vi "etapa2.vi"() -> ()   [LabVIEW 2017]
uses:
  <vilib>/Analysis/baseanly.llb/Mean (DBL).vi
  <vilib>/MakerHub/LINX/Public/Utilities/Open Serial.vi
  <vilib>/measure/maspectr.llb/FFT Spectrum (Mag-Phase) for 1 Chan.vi
  <vilib>/MakerHub/LINX/LMH-LINX.lvlib
  <vilib>/Analysis/NI_AALBase.lvlib
  <vilib>/measure/NI_MAPro.lvlib
panel:
  out "Frequência predominante (Hz)":dbl
  in  "Loop":u8
  in  "Janela":u8
  out "Frequências":cluster{"f0":dbl, "df":dbl, "magnitude":dbl[]}(graph)
  out "Pontos adquiridos":waveform(dbl)(graph)
  out "Dup Command Number":u16
  out "Tempo entre medidas":u8[](array[numeric])
  out "Device Name":string
  in  "Serial Port":refnum<visa-resource-name>="N/A"
  in  "Baud Rate Override":u32
  # "Aquisição"
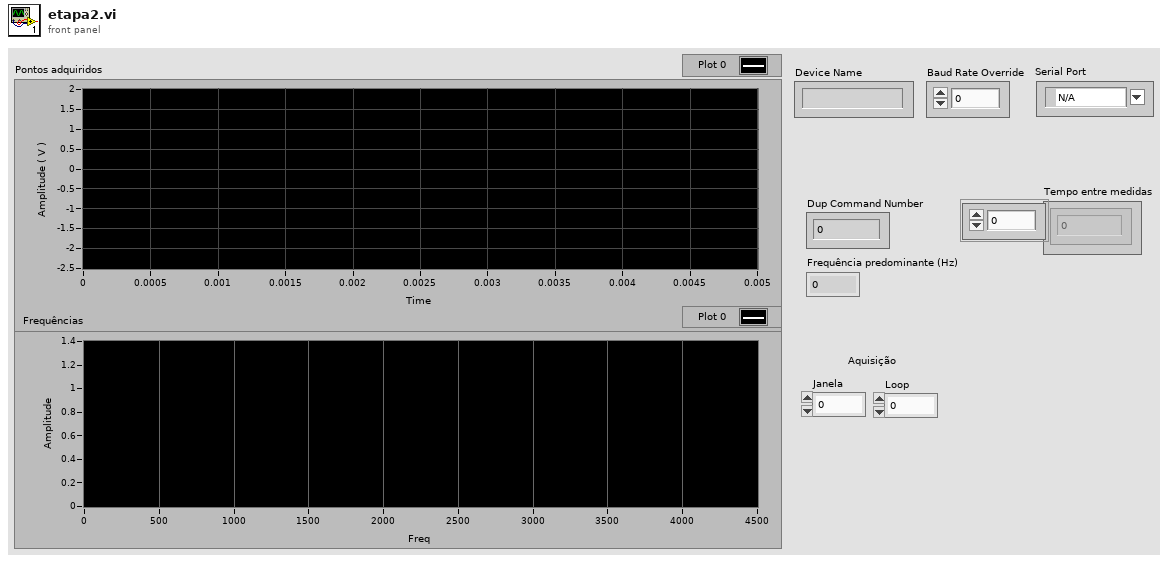
[diagram p1: front panel]
types:
  T1 = typedef "LMH-LINX.lvlib/LINX Ref.ctl" = cluster{"IO":T2, "Interface":T3, "LINX Device Config":T4}
  T2 = typedef "LMH-LINX.lvlib/Platform.ctl" = enum16{"Remote", "Local"}
  T3 = typedef "LMH-LINX.lvlib/Interface.ctl" = enum16{"Serial", "TCP"}
  T4 = typedef "LMH-LINX.lvlib/Device.lvlib/LINX Device Config.ctl" = cluster{"Interface":T3, "COM Port":refnum<visa-resource-name>, "TCP Configuration":T5, "Device Family":u8, "Device ID":u8, "Device Name":string, "TCP Ref":refnum<k5>, "Channels":T6}
  T5 = typedef "LMH-LINX.lvlib/Device.lvlib/TCP Config.ctl" = cluster{"IP Address":string, "Port":u16}
  T6 = typedef "LMH-LINX.lvlib/Channels.ctl" = cluster{"DI":u8[], "DO":u8[], "AI":u8[], "AO":u8[], "PWM":u8[], "QE":u8[], "UART":u8[], "I2C 2":u8[], "SPI":u8[], "CAN":u8[], "Servo":u8[], "AI Ref (V)":dbl, "AI Resolution (Bits)":u8, "AO Ref (V)":dbl, "AO Resolution (Bits)":u8}
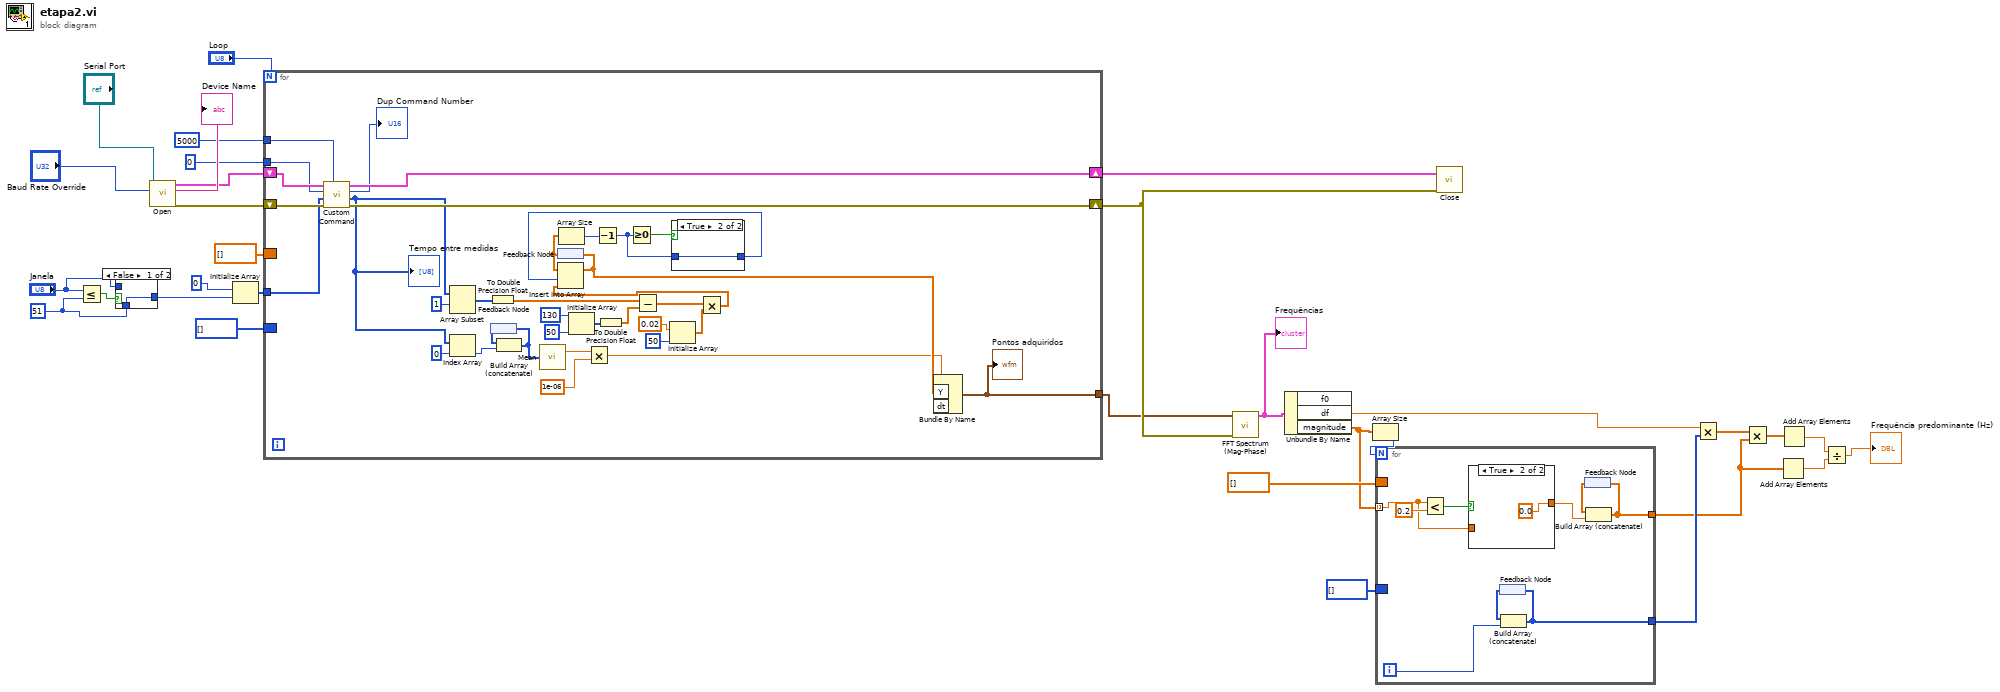
[diagram p0: block diagram]
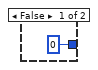
[diagram p4: hidden frame]
diagram:
  w16 = 51 ("y")
  n1 = Less Or Equal?(x="Janela", y=w16) -> (x <= y?=w21:bool)
  n2 = case shown="False" w21 {
    tunnel: "Janela" -> [_ w34]
    tunnel: [w33 w34] -> w19
    tunnel: w16 -> [w33 _]
    frame False {
    }
    frame True {
    }
  }
  n3 = call-poly <vilib>:"Open.vi"("Baud Rate Override"="Baud Rate Override", "Serial Port"="Serial Port") -> ("Error Out"=w27:errorcluster, "Device Name"=→"Device Name":string, "LINX Resource"=w29:T1)  [unwired: 7 in]
  n4 = Initialize Array(0 ("dimension size"), w19) -> (w17:i32[])
  n5 = for {
    N: "Loop" -> [_]
    tunnel: u16 0 ("Custom Command Number") -> [w68]
    tunnel: 5000 ("Timeout (100 ms)") -> [w64]
    shift-right: [w66] -> w26
    shift-left: w29 -> [w69]
    shift-right: [w65] -> w15
    shift-left: w27 -> [w67]
    border: dbl[] [] -> [_]
    border: u8[] [] -> [_]
    tunnel: w17 -> [w36]
    tunnel: [w35] -> w14
    n6 = call <vilib>:"Custom Command.vi"("Timeout (100 ms)"=w64, "Error In"=w67, "Data"=w36, "Custom Command Number"=w68, "LINX Resource"=w69) -> ("Error Out"=w65:errorcluster, "Response"=w61:u8[], "Dup Command Number"=→"Dup Command Number":u16, "LINX Resource"=w66:T1)  [unwired: 3 in]
    "Tempo entre medidas" <- w61
    n7 = Array Subset(array=w61, index=1) -> (w47:u8[])  [unwired: 1 in]
    n8 = Index Array(array=w61, index=0) -> (element=w59:u8)
    n9 = To Double Precision Float(number=w47) -> (double precision float=w46:dbl[])
    n10 = feedback #1() -> (w58:u8[])
    n11 = Build Array (concatenate)(w58, w59) -> (w57:u8[])
    n12 = feedback-in #1(w57) -> ()
    n13 = call-poly <vilib>:"Mean.vi"("X"=w57) -> ("mean"=w55:dbl)  [unwired: 1 out]
    n14 = feedback #2() -> (w52:dbl[])
    n15 = Array Size(array=w52) -> (size(s)=w51:i32)
    n16 = Initialize Array(130 ("element"), 50 ("dimension size")) -> (w44:i32[])
    n17 = Multiply(x=w55, y=1e-06) -> (x*y=w54:dbl)
    n18 = Decrement(x=w51) -> (x-1=w49:i32)
    n19 = To Double Precision Float(number=w44) -> (double precision float=w43:dbl[])
    n20 = Greater Or Equal To 0?(x=w49) -> (x >= 0?=w50:bool)
    n21 = Subtract(x=w46, y=w43) -> (x-y=w41:dbl[])
    n22 = Initialize Array(0.02 ("element"), 50 ("dimension size")) -> (w38:dbl[])
    n23 = case shown="True" w50 {
      tunnel: w49 -> [_ w71]
      tunnel: [0 w71] -> w48
      frame False {
      }
      frame True {
      }
    }
    n24 = Multiply(x=w41, y=w38) -> (x*y=w37:dbl[])
    n25 = Insert Into Array(array=w52, index=w48, new element=w37) -> (w56:dbl[])
    n26 = feedback-in #2(w56) -> ()
    n27 = Bundle By Name("Y"=w56, "dt"=w54) -> (w35:waveform(dbl))  [unwired: 1 in]
    "Pontos adquiridos" <- w35
  }
  n28 = call-poly <vilib>:"FFT Spectrum (Mag-Phase).vi"("error in (no error)"=w15, "time signal"=w14) -> ("magnitude"=w13:cluster{"f0":dbl, "df":dbl, "magnitude":dbl[]})  [unwired: 5 in, 4 out]
  "Frequências" <- w13
  n29 = Unbundle By Name(w13) -> ("df"=w10:dbl, "magnitude"=w3:dbl[])  [unwired: 1 out]
  n30 = Array Size(array=w3) -> (size(s)=w2:i32)
  n31 = for {
    N: w2 -> [_]
    tunnel: w3 -> [w77] mode=indexing
    border: dbl[] [] -> [_]
    tunnel: [w75] -> w7
    border: i32[] [] -> [_]
    tunnel: [w72] -> w11
    i -> [w73]
    n32 = Less?(x=w77, y=0.2) -> (x < y?=w79:bool)
    n33 = case shown="True" w79 {
      tunnel: [w81 0.0] -> w78
      tunnel: w77 -> [w81 _]
      frame False {
      }
      frame True {
      }
    }
    n34 = feedback #3() -> (w74:i32[])
    n35 = Build Array (concatenate)(w74, w73) -> (w72:i32[])
    n36 = feedback-in #3(w72) -> ()
    n37 = feedback #4() -> (w76:dbl[])
    n38 = Build Array (concatenate)(w76, w78) -> (w75:dbl[])
    n39 = feedback-in #4(w75) -> ()
  }
  n40 = call <vilib>:"Close.vi"("Error In"=w15, "LINX Resource"=w26) -> ()  [unwired: 9 in, 1 out]
  n41 = Multiply(x=w10, y=w11) -> (x*y=w9:dbl[])
  n42 = Multiply(x=w9, y=w7) -> (x*y=w8:dbl[])
  n43 = Add Array Elements(numeric array=w7) -> (sum=w5:dbl)
  n44 = Add Array Elements(numeric array=w8) -> (sum=w6:dbl)
  n45 = Divide(x=w6, y=w5) -> (x/y=→"Frequência predominante (Hz)":dbl)
